vi "Radians per Second to RPM (Scalar).vi"(3 "radians per second":dbl) -> (1 "rpm":dbl)   [LabVIEW 2017, in "NI_Robotics Utilities.lvlib"]
doc: "Converts an angular velocity from radians per second to rpm."
uses:
  <vilib>/robotics/Utilities/NI_Robotics Utilities.lvlib
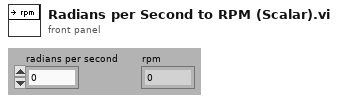
[diagram p1: front panel]
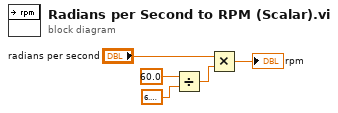
[diagram p0: block diagram]
diagram:
  n1 = Divide(x=60.0, y=6.283185307179586) -> (x/y=w4:dbl)
  n2 = Multiply(x="radians per second", y=w4) -> (x*y=→"rpm":dbl)
